vi "OP500Z8_ST5520_P.vi"(8 "errin":errorcluster, 10 "chemin de base":path, 11 "Refnum VISA en entrée":refnum<visa-resource-name>) -> (0 "error out":errorcluster caption="sortie d'erreur", 3 "R iso(MOhm)":dbl)   [LabVIEW 2020]
uses:
  Equipment/09 ST5520/Public/Lower/Config Measure/ST5520 Set Measurement Configuration.vi
  Equipment/09 ST5520/Public/Lower/Comparator/ST5520 Set Comparator.vi
  Equipment/09 ST5520/Public/Lower/Testing Status/ST5520 Start.vi
  Equipment/09 ST5520/Public/Lower/Testing Status/ST5520 State.vi
  VG/VG_Barre_Progression_ISO_P.vi
  Equipment/09 ST5520/Public/Lower/Measurement/ST5520 Read Resistance.vi
  Equipment/09 ST5520/Public/Lower/Testing Status/ST5520 Stop.vi
  <instrlib>/ST5520/ST5520.lvlib
panel:
  out "Glissière":u8(slide) scale=0.0..100.0
  out "Rin":string
  in  "lbl log std":string
  out "LOG STD":string
  out "LOG Html":string[](array[string])
  out "MSG":string
  out "PASS?":bool
  out "Status":T1(ring)
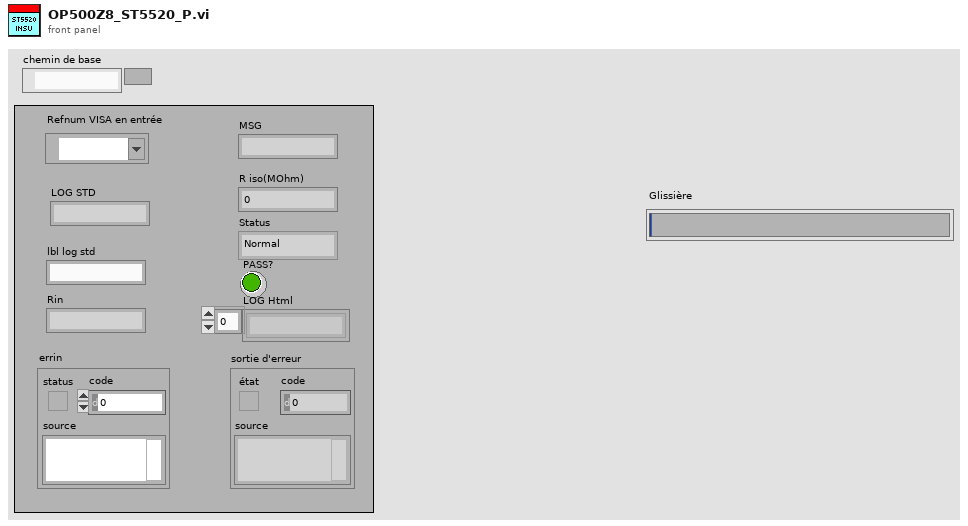
[diagram p1: front panel]
types:
  T1 = enum16{"Normal", "Over Flow", "Under Flow", "Error"}
  T2 = cluster{"Baud Rate":u32, "Frequency":enum8{"AUTO", "50", "60"}, "Resistance Range":cluster{"Range":enum16{"2M", "20M", "200M", "2000M", "4000M", "AUTO"}, "Set Check Range Change if AUTO":enum16{"ON", "OFF"}}, "Voltage":u16, "Timing":cluster{"Measurement Speed":enum16{"FAST", "SLOW"}, "Timer":cluster{"Set/Unset":enum8{"Set", "Unset"}, "Duration":dbl}, "Delay":cluster{"Set/Unset":enum8{"Set", "Unset"}, "Duration":dbl}}, "Beep":enum8{"PASS", "FAIL", "OFF", "END"}, "Mode":enum8{"CONTINUE", "PASSSTOP", "FAILSTOP", "SEQUENCE"}, "Upper Limit":cluster{"ON/OFF":enum8{"ON", "OFF"}, "Limit Value":dbl}, "Lower Limit":cluster{"ON/OFF":enum8{"ON", "OFF"}, "Limit Value":dbl}}
  T3 = cluster{"Range":enum16{"2M", "20M", "200M", "2000M", "4000M", "AUTO"}, "Set Check Range Change if AUTO":enum16{"ON", "OFF"}}
  T4 = cluster{"Measurement Speed":enum16{"FAST", "SLOW"}, "Timer":cluster{"Set/Unset":enum8{"Set", "Unset"}, "Duration":dbl}, "Delay":cluster{"Set/Unset":enum8{"Set", "Unset"}, "Duration":dbl}}
  T5 = enum8{"CONTINUE", "PASSSTOP", "FAILSTOP", "SEQUENCE"}
  T6 = cluster{"ON/OFF":enum8{"ON", "OFF"}, "Limit Value":dbl}
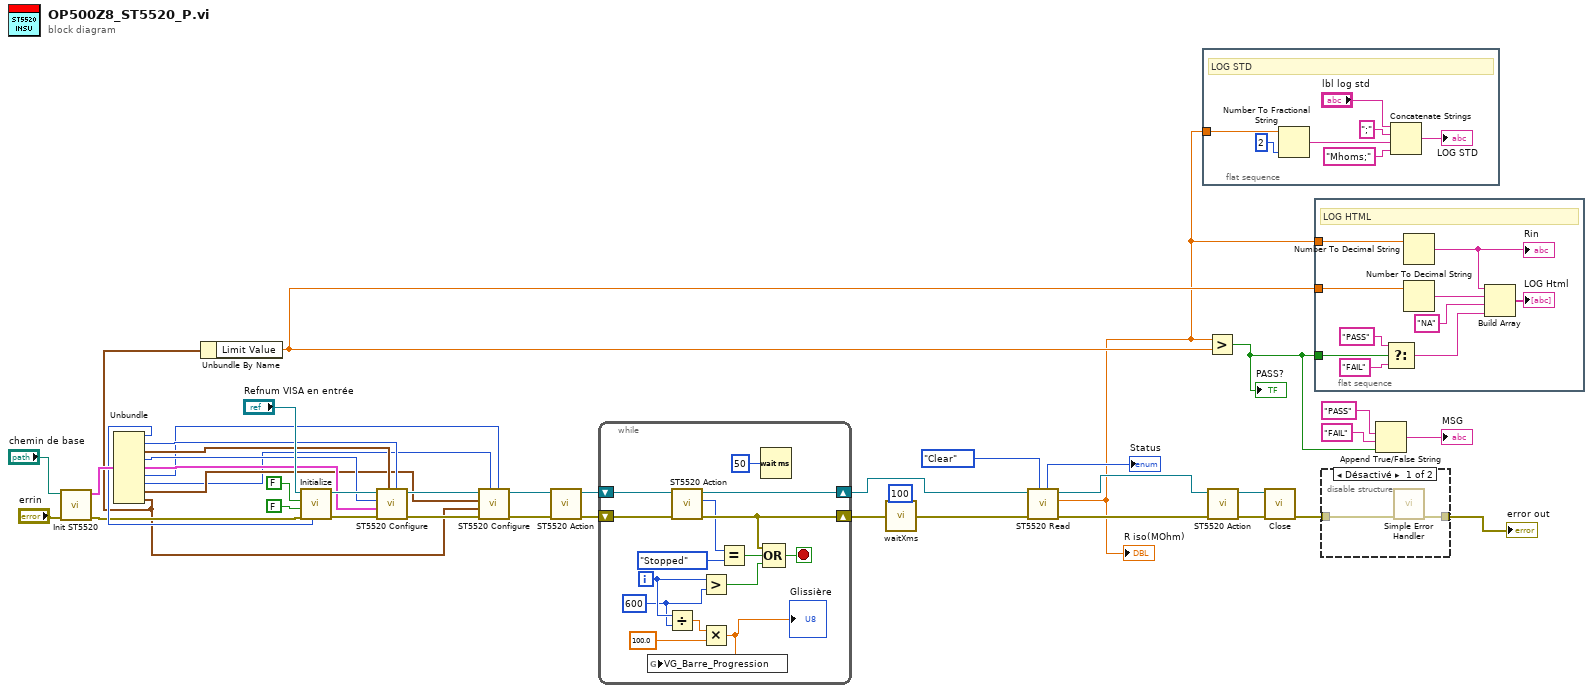
[diagram p0: block diagram]
diagram:
  n1 = call <userlib>:"Init ST5520.vi"("errin"="errin", "chemin de base"="chemin de base") -> ("error out"=w21:errorcluster, "Cluster Paramètres fichier Ini"=w24:T2)  [unwired: 8 in]
  n2 = Unbundle(w24) -> ("Baud Rate"=w23:u32, "Frequency"=w19:enum8{"AUTO", "50", "60"}, "Resistance Range"=w18:T3, "Voltage"=w20:u16, "Timing"=w17:T4, "Beep"=w14:enum8{"PASS", "FAIL", "OFF", "END"}, "Mode"=w15:T5, "Upper Limit"=w16:T6, "Lower Limit"=w13:T6)
  n3 = Unbundle By Name(w13) -> ("Limit Value"=w8:dbl)
  n4 = call <instrlib>:"Initialize.vi"("VISA resource name"="Refnum VISA en entrée", "ID Query (True)"=FALSE, "Reset (True)"=FALSE, "error in (no error)"=w21, "Baud Rate"=w23) -> ("VISA resource name out"=w28:refnum<visa-resource-name>, "error out"=w27:errorcluster)  [unwired: 4 in]
  n5 = call-poly "ST5520 Configure.vi"("Frequency"=w19, "Resistance Range"=w18, "error in (no error)"=w27, "Timing"=w17, "Voltage"=w20, "VISA resource name"=w28) -> ("error out"=w31:errorcluster, "VISA resource name out"=w29:refnum<visa-resource-name>)  [unwired: 4 in]
  n6 = call-poly "ST5520 Configure.vi"("Beep"=w14, "Mode"=w15, "error in (no error)"=w31, "Lower Limit"=w13, "Upper Limit"=w16, "VISA resource name"=w29) -> ("error out"=w32:errorcluster, "VISA resource name out"=w30:refnum<visa-resource-name>)  [unwired: 4 in]
  n7 = call-poly "ST5520 Action.vi"("error in (no error)"=w32, "VISA resource name"=w30) -> ("error out"=w36:errorcluster, "VISA resource name out"=w37:refnum<visa-resource-name>)  [unwired: 8 in]
  n8 = while {
    shift-right: [w57] -> w42
    shift-left: w37 -> [w54]
    shift-right: [w51] -> w6
    shift-left: w36 -> [w53]
    i -> [w47]
    stop <- w50 stop-if-true
    w46 = 600 ("y")
    n9 = Divide(x=w47, y=w46) -> (x/y=w45:dbl)
    n10 = call-poly "ST5520 Action.vi"("error in (no error)"=w53, "VISA resource name"=w54) -> ("error out"=w51:errorcluster, "State"=w48:enum8{"Stopped", "Testing ", "Discharging"}, "VISA resource name out"=w57:refnum<visa-resource-name>)  [unwired: 7 in]
    n11 = Greater?(x=w47, y=w46) -> (0:w49:bool)
    n12 = Multiply(x=w45, y=100.0) -> (x*y=w43:dbl)
    "Glissière" <- w43
    n13 = global write "VG_Barre_Progression_ISO_P.vi" "VG_Barre_Progression"(w43) -> ()
    n14 = Equal?(x=w48, y=enum8{"Stopped", "Testing ", "Discharging"}."Stopped" ("State")) -> (x = y?=w52:bool)
    n15 = Wait (ms)(milliseconds to wait=u32 50) -> ()  [unwired: 1 out]
    n16 = Compound Arithmetic op=OR(w51, w52, w49) -> (w50:bool)
  }
  n17 = call <userlib>:"waitXms.vi"("attente (ms)"=u32 100, "errin"=w6) -> ("errout"=w5:errorcluster)  [unwired: 13 in]
  n18 = call-poly "ST5520 Read.vi"("Clear Measurement"=enum16{"Remain", "Clear"}."Clear", "err in"=w5, "visa in"=w42) -> ("error out"=w38:errorcluster, "Measured Value (MOhm)"=w7:dbl, "VISA resource name out"=w39:refnum<visa-resource-name>, "Status"=→"Status":T1)  [unwired: 3 in, 2 out]
  "R iso(MOhm)" <- w7
  n19 = flat-sequence {
    tunnel: w7 -> [w61]
    frame #0 {
      # "LOG STD"
      n20 = Number To Fractional String(number=w61, precision (6)=i16 2 ("précision (6)")) -> (F-format string=w64:string)  [unwired: 2 in]
      n21 = Concatenate Strings("lbl log std", ";" ("chaîne"), w64, "Mhoms;" ("chaîne")) -> (→"LOG STD":string)
    }
  }
  n22 = Greater?(x=w7, y=w8) -> (0:w10:bool)
  "PASS?" <- w10
  n23 = call-poly "ST5520 Action.vi"("error in (no error)"=w38, "VISA resource name"=w39) -> ("error out"=w34:errorcluster, "VISA resource name out"=w35:refnum<visa-resource-name>)  [unwired: 8 in]
  n24 = call "Close.vi"("error in (no error)"=w34, "VISA resource name"=w35) -> ("error out"=w33:errorcluster)  [unwired: 9 in]
  n25 = flat-sequence {
    tunnel: w10 -> [w67]
    tunnel: w8 -> [w66]
    tunnel: w7 -> [w65]
    frame #0 {
      # "LOG HTML"
      n26 = Select(t="PASS", s=w67, f="FAIL") -> (s? t:f=w68:string)
      n27 = Number To Decimal String(number=w65) -> (decimal integer string=w74:string)  [unwired: 1 in]
      "Rin" <- w74
      n28 = Number To Decimal String(number=w66) -> (decimal integer string=w73:string)  [unwired: 1 in]
      n29 = Build Array(w74, w73, "NA" ("élément"), w68) -> (→"LOG Html":string[])
    }
  }
  n30 = disable-structure shown="Désactivé" {
    disable-tunnel: w33 -> [w76 w77]
    disable-tunnel: [w75 w77] -> w25
    frame Disabled {
      n31 = call <vilib>:"Simple Error Handler.vi"("error in (no error)"=w76) -> ("error out"=w75:errorcluster)  [unwired: 4 in, 4 out]
    }
    frame Enabled {
    }
  }
  "error out" <- w25
  n32 = Append True/False String(1:w10, 2:"FAIL" ("chaîne faux"), 3:"PASS" ("chaîne vrai")) -> (0:→"MSG":string)  [unwired: 1 in]
